vi "Read U16.vi"(8 "error in (no error)":errorcluster, 11 "Event in":refnum<class "Event U16.lvclass">) -> (0 "error out":errorcluster, 2 "U16":u16, 3 "Event out":refnum<class "Event U16.lvclass">)   [LabVIEW 2017, in "Event Actors.lvlib" / "Event U16.lvclass"]
uses:
  Event U16.lvclass
  Event U16.lvclass/Event U16.ctl
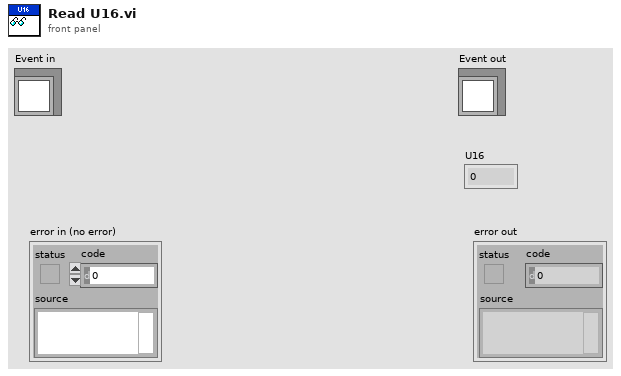
[diagram p1: front panel]
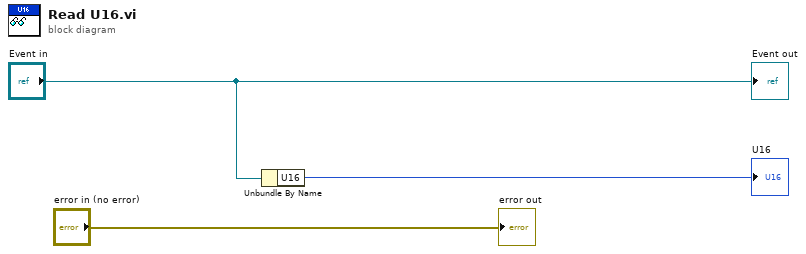
[diagram p0: block diagram]
diagram:
  n1 = Unbundle By Name("Event in") -> ("U16"=→"U16":u16)
  "Event out" <- "Event in"
  "error out" <- "error in (no error)"
